vi "ScriptReader.vi"(11 "Script File":path) -> (2 "Different Scripts":i32, 3 "Scripts":i32[][](array[numeric]))   [LabVIEW 2018]
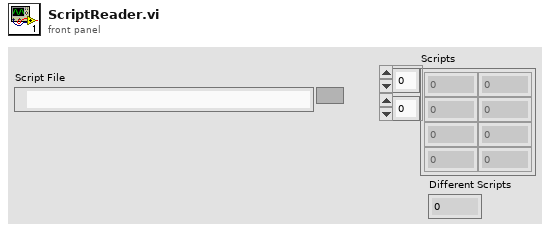
[diagram p1: front panel]
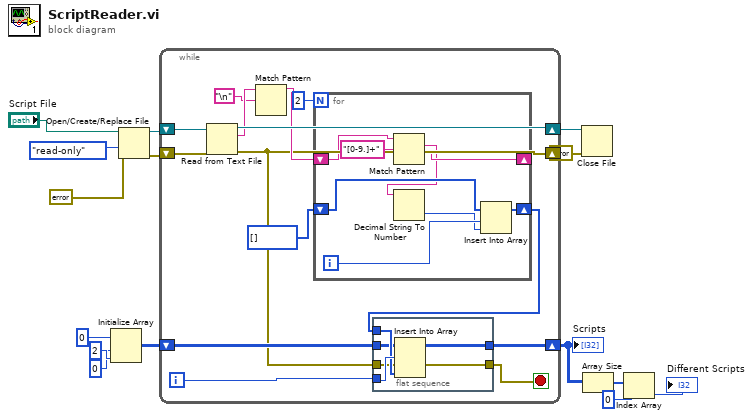
[diagram p0: block diagram]
diagram:
  n1 = Initialize Array(0 ("element"), 0 ("dimension size"), 2 ("dimension size")) -> (w8:i32[][])
  n2 = Open/Create/Replace File(file path (use dialog)="Script File", error in=errorcluster {"status"=FALSE, "code"=0, "source"=""}, access (0:read/write)=enum16{"read/write", "read-only", "write-only"}."read-only") -> (refnum out=w11:refnum<file>, error out=w10:errorcluster)  [unwired: 3 in, 1 out]
  n3 = while {
    shift-right: [w27] -> w14
    shift-left: w11 -> [w28]
    shift-right: [w17] -> _
    shift-left: w10 -> [w29]
    shift-right: [w19] -> w5
    shift-left: w8 -> [w18]
    i -> [w26]
    stop <- w16 stop-if-true
    n4 = Read from Text File(file (use dialog)=w28, error in=w29) -> (refnum out=w27:refnum<file>, text=w25:string, error out=w17:errorcluster)  [unwired: 2 in, 1 out]
    n5 = Match Pattern(string=w25, regular expression="\n") -> (before substring=w21:string)  [unwired: 1 in, 3 out]
    n6 = for {
      N: 2 -> [_]
      shift-right: [w40] -> _
      shift-left: w21 -> [w42]
      shift-right: [w35] -> w20
      shift-left: i32[] [] -> [w37]
      i -> [w39]
      n7 = Match Pattern(string=w42, regular expression="[0-9.]+") -> (match substring=w36:string, after substring=w40:string)  [unwired: 1 in, 2 out]
      n8 = Decimal String To Number(string=w36) -> (number=w38:i32)  [unwired: 2 in, 1 out]
      n9 = Insert Into Array(array=w37, index=w39, new element=w38) -> (w35:i32[])
    }
    n10 = flat-sequence {
      tunnel: w26 -> [w34]
      tunnel: w20 -> [w33]
      tunnel: [w32] -> w19
      tunnel: w18 -> [w31]
      tunnel: w17 -> [w30]
      tunnel: [w30] -> w16
      frame #0 {
        n11 = Insert Into Array(array=w31, index (row)=w34, new element=w33) -> (w32:i32[][])  [unwired: 1 in]
      }
    }
  }
  "Scripts" <- w5
  n12 = Close File(refnum=w14, error in=errorcluster {"status"=FALSE, "code"=0, "source"=""}) -> ()  [unwired: 2 out]
  n13 = Array Size(array=w5) -> (size(s)=w3:i32[])
  n14 = Index Array(array=w3, index=0) -> (element=→"Different Scripts":i32)
